vi "KH Control.vi"(8 "error in":errorcluster, 11 "Channel Setting":T1(array[cluster])=[{"Channel"=enum."Channel 1", "Gain"=enum."1000x", "Shunt Resistor"=enum."50 Ohms", "Measure"=enum."Current(Diff)"}, {"Channel"=enum."Channel 2", "Gain"=enum."1000x", "Shunt Resistor"=enum."50k Ohms", "Measure"=enum."Current(Diff)"}, {"Channel"=enum."Channel 3", "Gain"=enum."1000x", "Shunt Resistor"=enum."50 Ohms", "Measure"=enum."Voltage(SE+)"}, {"Channel"=enum."Channel 4", "Gain"=enum."1000x", "Shunt Resistor"=enum."50 Ohms", "Measure"=enum."Voltage(SE+)"}, {"Channel"=enum."Channel 5", "Gain"=enum."1000x", "Shunt Resistor"=enum."50 Ohms", "Measure"=enum."Voltage(SE+)"}, {"Channel"=enum."Channel 6", "Gain"=enum."1000x", "Shunt Resistor"=enum."50k Ohms", "Measure"=enum."Current(Diff)"}, {"Channel"=enum."Channel 7", "Gain"=enum."1000x", "Shunt Resistor"=enum."50 Ohms", "Measure"=enum."Voltage(SE+)"}, {"Channel"=enum."Channel 8", "Gain"=enum."1000x", "Shunt Resistor"=enum."50k Ohms", "Measure"=enum."Current(Diff)"}]) -> (0 "error out":errorcluster)   [LabVIEW 2013]
panel:
  in  "VISA Refnum in":refnum<visa-resource-name>="COM3"
  # "1. Create a copy of drivers under C:\\Krohn-Hite 7008\\Drivers if there is none. \n2. In device manager browse the driver for Krohn-Hite"
  # "Measure Current: Current, Shunt Resistor: 50kOhm\nMeasure Voltage: Voltage, Shunt Resistor: Open\nApplying Gate: Current, Shunt Resistor: 50kOhm\n                      Open all the unused gate"
  # "Warning: repeated channels will cause false reading in the lock-in"
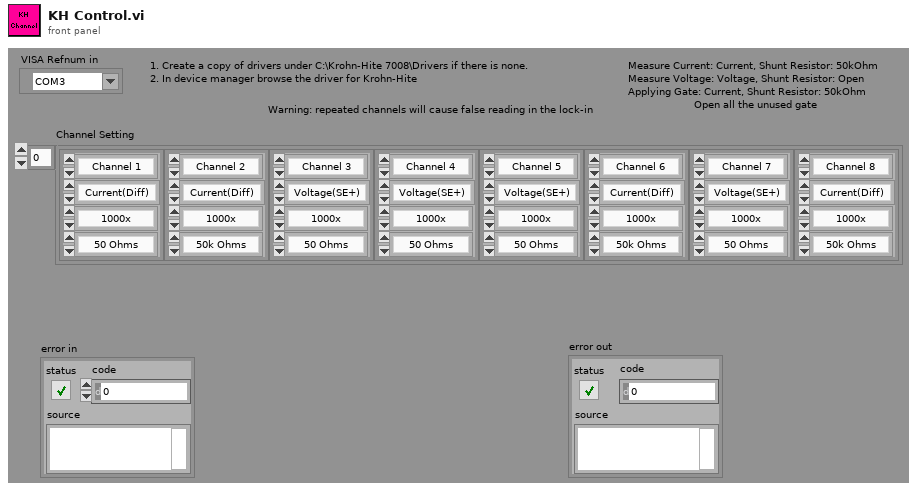
[diagram p1: front panel]
types:
  T1 = cluster{"Channel":enum16{"Channel 1", "Channel 2", "Channel 3", "Channel 4", "Channel 5", "Channel 6", "Channel 7", "Channel 8"}, "Gain":enum16{"1x", "10x", "100x", "1000x"}, "Shunt Resistor":enum16{"Open", "50 Ohms", "500 Ohms", "5k Ohms", "50k Ohms"}, "Measure":enum16{"Float", "Current(Diff)", "Voltage(SE+)"}}[]
  T2 = enum16{"Channel 1", "Channel 2", "Channel 3", "Channel 4", "Channel 5", "Channel 6", "Channel 7", "Channel 8"}
  T3 = enum16{"Open", "50 Ohms", "500 Ohms", "5k Ohms", "50k Ohms"}
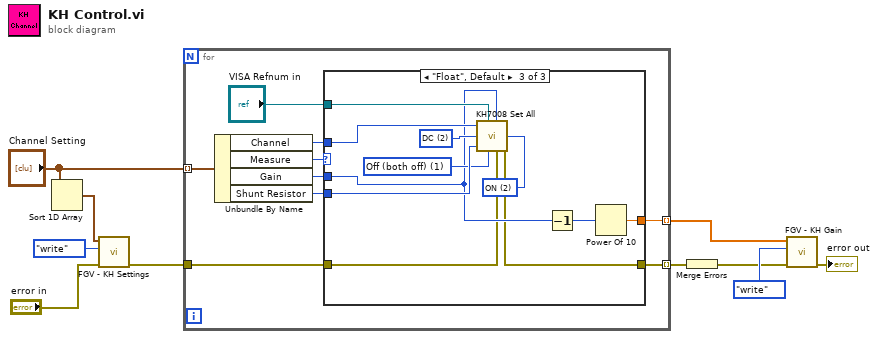
[diagram p0: block diagram]
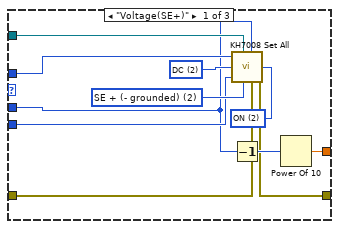
[diagram p2: hidden frame]
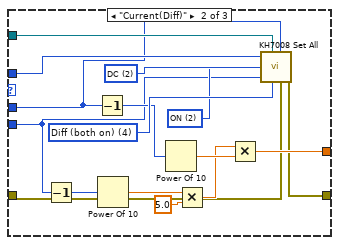
[diagram p3: hidden frame]
diagram:
  n1 = Sort 1D Array(array="Channel Setting") -> (sorted array=w10:T1)
  n2 = call "FGV - KH Settings.vi"("error in"="error in", "Function"=enum16{"write", "read"}."write", "Channel Setting"=w10) -> ("error out"=w5:errorcluster)  [unwired: 3 in, 1 out]
  n3 = for {
    tunnel: "Channel Setting" -> [w15] mode=indexing
    tunnel: [w13] -> w8 mode=indexing
    tunnel: w5 -> [w12]
    tunnel: [w11] -> w4 mode=indexing
    n4 = Unbundle By Name(w15) -> ("Channel"=w18:T2, "Measure"=w14:enum16{"Float", "Current(Diff)", "Voltage(SE+)"}, "Gain"=w17:enum16{"1x", "10x", "100x", "1000x"}, "Shunt Resistor"=w16:T3)
    n5 = case shown="\"Float\", Default" w14 {
      tunnel: w18 -> [w27 w46 w57]
      tunnel: w17 -> [w23 w39 w50]
      tunnel: w16 -> [w26 w33 w55]
      tunnel: "VISA Refnum in" -> [w25 w42 w52]
      tunnel: [w22 w41 w49] -> w13
      tunnel: w12 -> [w21 w32 w48]
      tunnel: [w20 w31 w47] -> w11
      frame "Voltage(SE+)" {
        w28 = u16 2 items=["Off (both off)"=1, "SE + (- grounded)"=2, "SE - (+ grounded)"=3, "Diff (both on)"=4] ("Input Coupling")
        w29 = u16 2 items=["OFF"=1, "ON"=2] ("Bandwidth Filter")
        w30 = u16 2 items=["AC"=1, "DC"=2] ("Coupling")
        n6 = call "KH7008 Set All.vi"("Channel"=w27, "VISA Refnum in"=w25, "Coupling"=w30, "Shunt Resistor"=w26, "Input Coupling"=w28, "Gain"=w23, "Bandwidth Filter"=w29, "error in (no error)"=w21) -> ("error out"=w20:errorcluster)  [unwired: 1 in]
        n7 = Decrement(x=w23) -> (x-1=w24:enum16{"1x", "10x", "100x", "1000x"})
        n8 = Power Of 10(x=w24) -> (10^x=w22:dbl)
      }
      frame "Current(Diff)" {
        w43 = u16 2 items=["OFF"=1, "ON"=2] ("Bandwidth Filter")
        w44 = u16 4 items=["Off (both off)"=1, "SE + (- grounded)"=2, "SE - (+ grounded)"=3, "Diff (both on)"=4] ("Input Coupling")
        w45 = u16 2 items=["AC"=1, "DC"=2] ("Coupling")
        n9 = Decrement(x=w33) -> (x-1=w34:T3)
        n10 = Decrement(x=w39) -> (x-1=w40:enum16{"1x", "10x", "100x", "1000x"})
        n11 = Power Of 10(x=w34) -> (10^x=w36:dbl)
        n12 = Power Of 10(x=w40) -> (10^x=w38:dbl)
        n13 = Multiply(x=w36, y=5.0) -> (x*y=w35:dbl)
        n14 = Multiply(x=w35, y=w38) -> (x*y=w41:dbl)
        n15 = call "KH7008 Set All.vi"("Channel"=w46, "VISA Refnum in"=w42, "Coupling"=w45, "Shunt Resistor"=w33, "Input Coupling"=w44, "Gain"=w39, "Bandwidth Filter"=w43, "error in (no error)"=w32) -> ("error out"=w31:errorcluster)  [unwired: 1 in]
      }
      frame "Float", Default {
        w53 = u16 2 items=["OFF"=1, "ON"=2] ("Bandwidth Filter")
        w54 = u16 1 items=["Off (both off)"=1, "SE + (- grounded)"=2, "SE - (+ grounded)"=3, "Diff (both on)"=4] ("Input Coupling")
        w56 = u16 2 items=["AC"=1, "DC"=2] ("Coupling")
        n16 = call "KH7008 Set All.vi"("Channel"=w57, "VISA Refnum in"=w52, "Coupling"=w56, "Shunt Resistor"=w55, "Input Coupling"=w54, "Gain"=w50, "Bandwidth Filter"=w53, "error in (no error)"=w48) -> ("error out"=w47:errorcluster)  [unwired: 1 in]
        n17 = Decrement(x=w50) -> (x-1=w51:enum16{"1x", "10x", "100x", "1000x"})
        n18 = Power Of 10(x=w51) -> (10^x=w49:dbl)
      }
    }
  }
  n19 = Merge Errors(w4) -> (w3:errorcluster)
  n20 = call <userlib>:"FGV - KH Gain.vi"("error in"=w3, "Function"=enum16{"write", "read"}."write", "Array"=w8) -> ("error out"=→"error out":errorcluster)  [unwired: 3 in, 1 out]
